vi "Read Pump Control Value.vi"(8 "error in":errorcluster, 11 "CPC in":refnum<class "3022A.lvclass">) -> (0 "error out":errorcluster, 2 "Val":u8, 3 "CPC out":refnum<class "3022A.lvclass">)   [LabVIEW 2014, in "3022A.lvclass"]
uses:
  3022A/3022A.lvclass
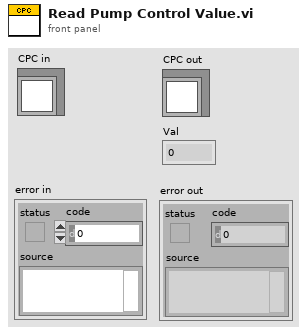
[diagram p1: front panel]
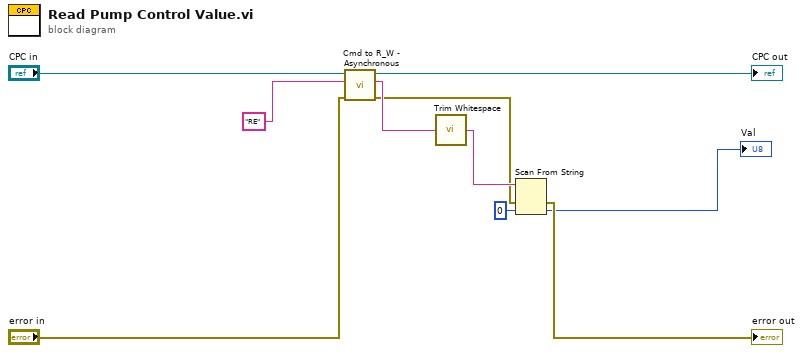
[diagram p0: block diagram]
diagram:
  n1 = call-dynamic "Cmd to R_W - Asynchronous.vi"("error in"="error in", "write buffer"="RE" ("string"), "Serial IO in"="CPC in") -> ("error out"=w2:errorcluster, "read buffer"=w4:string, "Serial IO out"=→"CPC out":refnum<class "3022A.lvclass">)  [unwired: 6 in]
  n2 = call <vilib>:"Trim Whitespace.vi"("string"=w4) -> ("trimmed string"=w3:string)  [unwired: 1 in]
  n3 = Scan From String(input string=w3, error in=w2, default 1=u8 0 ("default value 1")) -> (error out=→"error out":errorcluster, output 1=→"Val":u8)  [unwired: 2 in, 2 out]
